vi "Reference Queue (Multiple Messages).vi"   [LabVIEW 2019, in "Message Queue.lvlib"]
doc: "Function to enqueue a Message in a Queue of other Module."
uses:
  Message Queue.lvlib
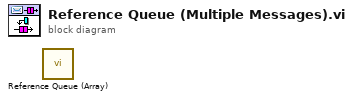
[diagram p0: block diagram]
diagram:
  n1 = call "Reference Queue (Array).vi"() -> ()  [unwired: 11 in, 1 out]
